vi "Write User File (SubVI).vi"(0 "configuration file path":path=path "C:/Projet_CETAL_DESY_CSCI/POSTES LOCAUX/PROJECT_GAIA_HP/Development/Config/User.ini" caption="chemin du fichier de configuration", 1 "User file contents Watlow":dbl[](array[numeric]) format="%#.3g", 7 "error in (no error)":errorcluster caption="entrée d'erreur (pas d'erreur)") -> (24 "error?":bool caption="erreur ?", 27 "error out":errorcluster caption="sortie d'erreur")   [LabVIEW 2017]
uses:
  <vilib>/Utility/config.llb/Write Key (String).vi
  <vilib>/Utility/config.llb/NI_LVConfig.lvlib
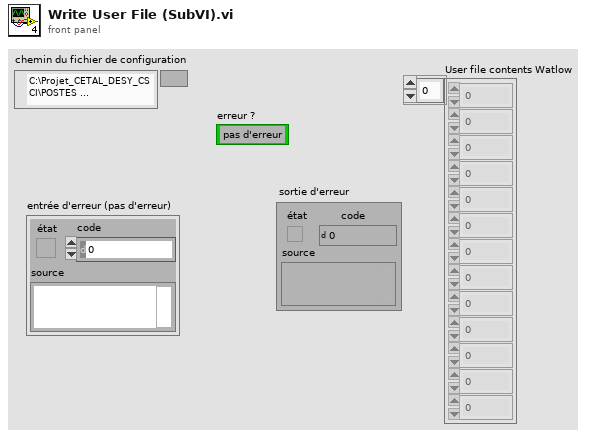
[diagram p1: front panel]
types:
  T1 = typedef "NI_LVConfig.lvlib/Config Data RefNum.ctl" = refnum<k1>
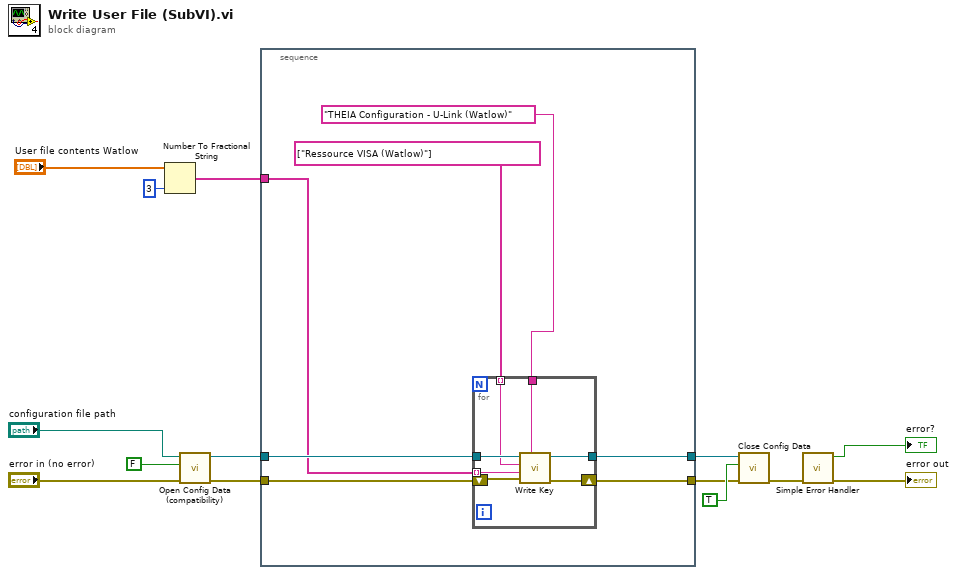
[diagram p0: block diagram]
diagram:
  n1 = Number To Fractional String(number="User file contents Watlow", precision (6)=i16 3) -> (F-format string=w4:string[])  [unwired: 2 in]
  n2 = call <vilib>:"Open Config Data (compatibility).vi"("error in (no error)"="error in (no error)", "create file if necessary (T)"=FALSE ("create file if necessary? (T)"), "configuration file path"="configuration file path") -> ("error out"=w13:errorcluster, "refnum"=w8:T1)  [unwired: 6 in, 1 out]
  n3 = stacked-sequence {
    tunnel: w13 -> [w21]
    tunnel: w8 -> [w20]
    tunnel: w4 -> [w19]
    tunnel: [w16] -> w2
    tunnel: [w15] -> w1
    frame #0 {
      n4 = for {
        shift-right: [w27] -> w16
        shift-left: w21 -> [w28]
        tunnel: w20 -> [w26]
        tunnel: w19 -> [w25] mode=indexing
        tunnel: string[] ["Ressource VISA (Watlow)"] -> [w24] mode=indexing
        tunnel: "THEIA Configuration - U-Link (Watlow)" ("section") -> [w23]
        tunnel: [w22] -> w15
        n5 = call-poly <vilib>:"Write Key.vi"("section"=w23, "error in (no error)"=w28, "value"=w25, "key"=w24, "refnum"=w26) -> ("error out"=w27:errorcluster, "refnum out"=w22:T1)  [unwired: 4 in, 1 out]
      }
    }
  }
  n6 = call <vilib>:"Close Config Data.vi"("error in (no error)"=w2, "write file if changed (T)"=TRUE ("write configuration file? (T)"), "refnum"=w1) -> ("error out"=w12:errorcluster)  [unwired: 8 out]
  n7 = call <vilib>:"Simple Error Handler.vi"("error in (no error)"=w12) -> ("error?"=→"error?":bool, "error out"=→"error out":errorcluster)  [unwired: 1 in, 6 out]
